vi "Open Connection.vi"(8 "error in (no error)":errorcluster, 9 "connection timeout (15)":i32=10, 10 "ConnectionString":string, 11 "HostDB in":refnum<class "SQLite.lvclass">) -> (0 "error out":errorcluster, 3 "HostDB out":refnum<class "SQLite.lvclass">)   [LabVIEW 2021, in "SQLite.lvclass"]
uses:
  SQLite.lvclass
  SQLite.lvclass/SQLite.ctl
  <vilib>/drjdpowell/SQLite Library/SQL Connection/Open (string).vi
  <vilib>/drjdpowell/SQLite Library/SQL Connection/Connection.lvclass
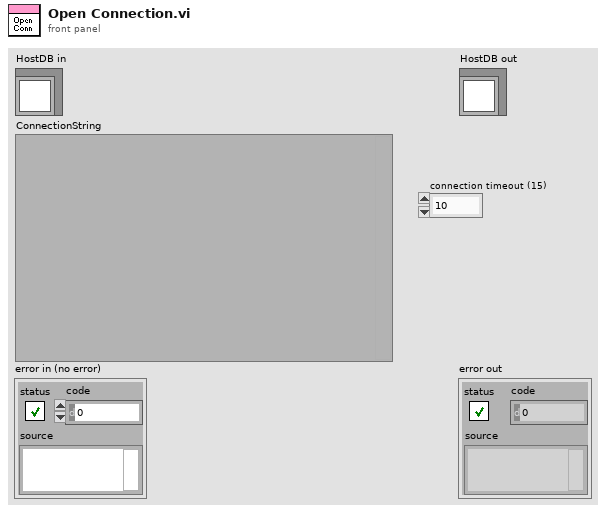
[diagram p1: front panel]
types:
  T1 = enum16{"New or existing", "Existing", "Read only"}
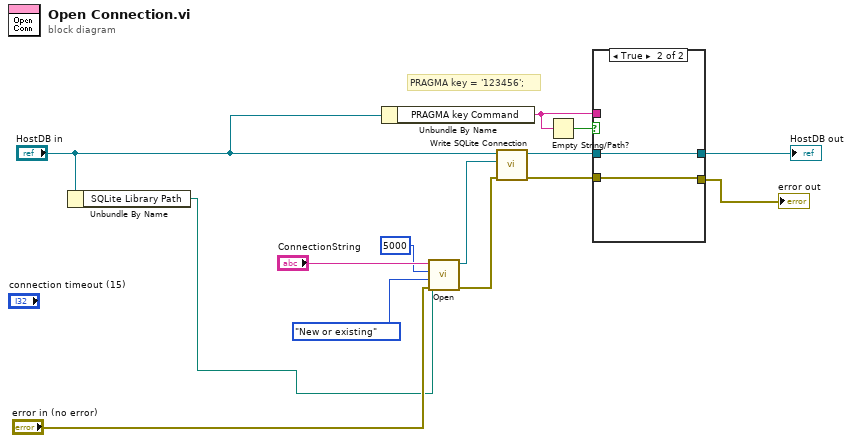
[diagram p0: block diagram]
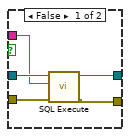
[diagram p2: hidden frame]
diagram:
  # "PRAGMA key = '123456';"
  n1 = Unbundle By Name("HostDB in") -> ("SQLite Library Path"=w1:path)
  n2 = Unbundle By Name("HostDB in") -> ("PRAGMA key Command"=w6:string)
  n3 = call-poly <vilib>:"Open.vi"("SQLite Library Path"=w1, "error in (no error)"="error in (no error)", "File Option"=T1."New or existing", "busy timeout (ms)"=5000, "db file"="ConnectionString") -> ("error out"=w13:errorcluster, "SQLite Connection"=w14:refnum<class "Connection.lvclass">)  [unwired: 5 in]
  n4 = call-dynamic "Write SQLite Connection.vi"("error in (no error)"=w13, "SQLite.lvlib:Connection"=w14, "SQLite in"="HostDB in") -> ("error out"=w4:errorcluster, "SQLite out"=w8:refnum<class "SQLite.lvclass">)  [unwired: 7 in]
  n5 = Empty String/Path?(string/path=w6) -> (empty?=w5:bool)
  n6 = case shown="True" w5 {
    tunnel: w8 -> [w19 w21]
    tunnel: [w18 w21] -> w7
    tunnel: w6 -> [w17 _]
    tunnel: w4 -> [w16 w20]
    tunnel: [w15 w20] -> w3
    frame False {
      n7 = call-dynamic "SQL Execute.vi"("error in (no error)"=w16, "Command Text"=w17, "HostDB in"=w19) -> ("error out"=w15:errorcluster, "HostDB out"=w18:refnum<class "SQLite.lvclass">)  [unwired: 4 in, 3 out]
    }
    frame True {
    }
  }
  "error out" <- w3
  "HostDB out" <- w7
